vi "Ctor.vi"(8 "error in (no error)":errorcluster, 11 "Team Dashboard Panel in":refnum<class "Team Dashboard Panel.lvclass">) -> (0 "error out":errorcluster, 3 "Team Dashboard Panel out":refnum<class "Team Dashboard Panel.lvclass">)   [LabVIEW 2020, in "SB App.lvlib" / "Team Dashboard Panel.lvclass"]
uses:
  Team Dashboard Panel.lvclass
  Team Status Data.ctl
  SquareBattle/Team Stats.ctl
  SquareBattle/Team State.ctl
  Team Dashboard Panel.lvclass/Team Dashboard Panel.ctl
  <vilib>/IlluminatedG/IG OOPanel/OOPanel/ArrayPanel/ArrayPanel.lvclass
  SquareBattle/SquareBattle.lvlib
  SB App.lvlib
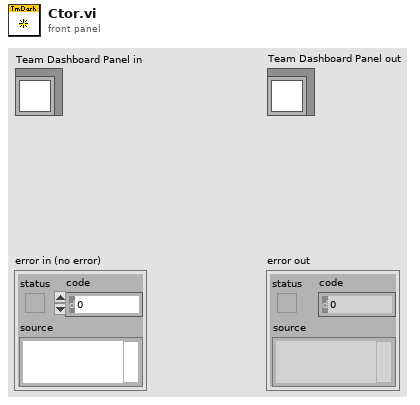
[diagram p1: front panel]
types:
  T1 = typedef "SquareBattle.lvlib/Team Stats.ctl" = cluster{"Squares":i32, "Generated":i32, "Kills":i32, "Eliminated":i32, "Collisions":i32}
  T2 = typedef "SB App.lvlib/Team Status Data.ctl" = cluster{"Team Stats":T1, "Team State":T3}
  T3 = typedef "SquareBattle.lvlib/Team State.ctl" = enum16{"Active", "Defeated", "Won"}
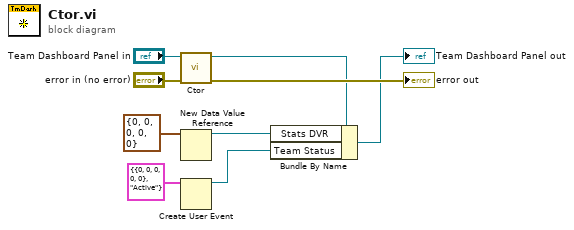
[diagram p0: block diagram]
diagram:
  n1 = call-parent "Ctor.vi"("error in (no error)"="error in (no error)", "ArrayPanel in"="Team Dashboard Panel in") -> ("error out"=→"error out":errorcluster, "ArrayPanel out"=w4:refnum<class "Team Dashboard Panel.lvclass">)  [unwired: 8 in]
  n2 = New Data Value Reference(data value=T1 {"Squares"=0, "Generated"=0, "Kills"=0, "Eliminated"=0, "Collisions"=0} ("Team Stats")) -> (data value reference=w1:refnum<data-value>)  [unwired: 1 in, 1 out]
  n3 = Create User Event(user event datatype=T2 {"Team Stats"={"Squares"=0, "Generated"=0, "Kills"=0, "Eliminated"=0, "Collisions"=0}, "Team State"=enum."Active"} ("Team Status Data")) -> (user event=w5:refnum<user-event>)  [unwired: 1 in, 1 out]
  n4 = Bundle By Name(cluster=w4, "Stats DVR"=w1, "Team Status"=w5) -> (→"Team Dashboard Panel out":refnum<class "Team Dashboard Panel.lvclass">)
